vi "GetType.vi"(8 "error in (no error)":errorcluster, 11 "Configure Channel Msg in":refnum<class "Configure Channel Msg.lvclass">) -> (0 "error out":errorcluster, 2 "Data Sample":variant, 3 "Configure Channel Msg out":refnum<class "Configure Channel Msg.lvclass">)   [LabVIEW 2014, in "CS++Scope.lvlib" / "Configure Channel Msg.lvclass"]
doc: "This VI delivers a sample of the data type format the message expects."
uses:
  Configure Channel Msg.lvclass
  Configure Channel Msg.lvclass/Configure Channel Msg.ctl
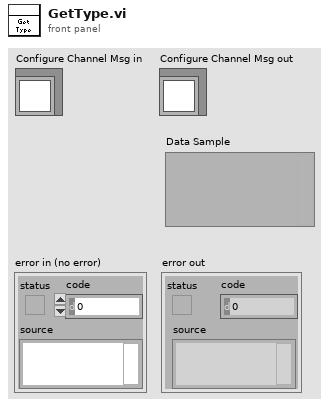
[diagram p1: front panel]
types:
  T1 = cluster{"channel name (\"CHANNEL1\")":string, "probe attenuation (1:1.0)":dbl, "vertical range (10.0 V)":dbl[unit], "vertical offset (0.0 V)":dbl[unit], "channel enabled (True)":bool, "vertical coupling (DC)":i32}
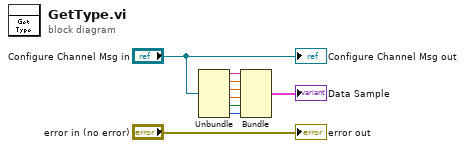
[diagram p0: block diagram]
diagram:
  n1 = Unbundle("Configure Channel Msg in") -> (w7:string, w6:dbl, w5:dbl[unit], w4:dbl[unit], w3:bool, w2:i32)
  n2 = Bundle("channel name (\"CHANNEL1\")"=w7, "probe attenuation (1:1.0)"=w6, "vertical range (10.0 V)"=w5, "vertical offset (0.0 V)"=w4, "channel enabled (True)"=w3, "vertical coupling (DC)"=w2) -> (→"Data Sample":T1)  [unwired: 1 in]
  "error out" <- "error in (no error)"
  "Configure Channel Msg out" <- "Configure Channel Msg in"
